vi "Backpressure Test.vi"() -> ()   [LabVIEW 2021]
uses:
  TypeDefs/Write Configuration.ctl
  TypeDefs/Read Configuration.ctl
  TypeDefs/Read Position.ctl
  TypeDefs/Data Element Details.ctl
  57e1f68e-aac2-4a5b-aa1d-bebc566d32eb.vi
  9744b0b2-8e27-4e4b-9bb7-f1c9ce8a1c96.vi
  07aec1d7-8ce0-4024-a95f-672f00c3de72.vi
  4385ff32-2761-4e03-bb1f-28e6c483433c.vi
  f7503771-80fd-45f4-b74f-3b2e92972461.vi
  c45c08b2-ea76-45d8-bd4a-0684d2e8d800.vi
  7eb9dc38-34d0-42a6-b102-5ea04e06049c.vi
  4e7c2fe8-0442-4db9-92fd-a364be716cb9.vi
  4ed2d6ae-5cba-444e-b9a2-7f82c0cf321a.vi
  ad8698de-81cd-4e11-8f1e-14e550fbdb4f.vi
  5ece5910-7f94-4528-9bc0-c785044b768d.vi
  f9d3fdbb-ee3c-4ad5-adeb-5751b16ba1b5.vi
  27686e40-44d3-4caa-b17a-767073325966.vi
  2cbba55c-0004-4c00-ad5c-760cc39579e2.vi
  0906a7d2-1e19-4f35-b09e-2fcf277513f2.vi
  7f108e34-9106-4d76-aec0-60a0699c295a.vi
  d49a2fac-eb09-4004-8c8e-5ff393d47214.vi
  3aa2fef3-6e97-4fad-b2b2-b9e5007bd319.vi
  66206acd-3047-480d-a13c-978b6dcd533f.vi
  a2f45c90-3ccc-4f15-aad7-08559cb123ac.vi
  32cec7b8-6370-43d4-931e-f60ddee9201a.vi
  63e088bb-fba7-44f9-b616-fb479035f017.vi
  b43ac5ef-eb88-421e-b33d-2ede57dd7442.vi
  e418e56f-4089-412c-bbf8-0d1a0f138b1a.vi
  e25f8ffa-7016-4157-92d2-29af65897e26.vi
  5e39a1b3-a940-464c-8f68-1595816f1c00.vi
  ac948e10-57ad-454e-bb7c-9577dd8c26ef.vi
  ffa58009-d41b-421a-8cf9-7a707b687784.vi
  8f16d32d-2386-471b-852e-c92f1fa65af2.vi
  57e1f68e-aac2-4a5b-aa1d-bebc566d32eb.vi/49b3dd2d-4579-4089-b72e-3f0875c862f2.vi
  SubVIs/Check Error.vi
  57e1f68e-aac2-4a5b-aa1d-bebc566d32eb.vi/1e2c93d0-55b0-4d6c-a9da-21395a664279.vi
  SubVIs/Get Backpressure Name.vi
  57e1f68e-aac2-4a5b-aa1d-bebc566d32eb.vi/7bb13226-97f3-4dcb-9346-06ec631a2876.vi
  SubVIs/Get dll Path.vi
  9744b0b2-8e27-4e4b-9bb7-f1c9ce8a1c96.vi/59915726-1e10-4578-8453-be1b9fd8d311.vi
  9744b0b2-8e27-4e4b-9bb7-f1c9ce8a1c96.vi/331f6ecb-7ec4-4931-b93d-4fbd8d66a851.vi
  07aec1d7-8ce0-4024-a95f-672f00c3de72.vi/3d5c1244-b460-4622-96d1-ee1e369932ac.vi
  Utilities/Get Size.vi
  07aec1d7-8ce0-4024-a95f-672f00c3de72.vi/b3361ac9-0b85-4d75-8feb-76d028d0c03f.vi
  SubVIs/Get Element Write Position.vi
  SubVIs/Notify Of New Write.vi
  f7503771-80fd-45f4-b74f-3b2e92972461.vi/49b3dd2d-4579-4089-b72e-3f0875c862f2.vi
  f7503771-80fd-45f4-b74f-3b2e92972461.vi/1e2c93d0-55b0-4d6c-a9da-21395a664279.vi
  f7503771-80fd-45f4-b74f-3b2e92972461.vi/7bb13226-97f3-4dcb-9346-06ec631a2876.vi
  c45c08b2-ea76-45d8-bd4a-0684d2e8d800.vi/59915726-1e10-4578-8453-be1b9fd8d311.vi
  c45c08b2-ea76-45d8-bd4a-0684d2e8d800.vi/331f6ecb-7ec4-4931-b93d-4fbd8d66a851.vi
  7eb9dc38-34d0-42a6-b102-5ea04e06049c.vi/3d5c1244-b460-4622-96d1-ee1e369932ac.vi
  7eb9dc38-34d0-42a6-b102-5ea04e06049c.vi/b3361ac9-0b85-4d75-8feb-76d028d0c03f.vi
  4ed2d6ae-5cba-444e-b9a2-7f82c0cf321a.vi/49b3dd2d-4579-4089-b72e-3f0875c862f2.vi
  4ed2d6ae-5cba-444e-b9a2-7f82c0cf321a.vi/1e2c93d0-55b0-4d6c-a9da-21395a664279.vi
  4ed2d6ae-5cba-444e-b9a2-7f82c0cf321a.vi/7bb13226-97f3-4dcb-9346-06ec631a2876.vi
  ad8698de-81cd-4e11-8f1e-14e550fbdb4f.vi/59915726-1e10-4578-8453-be1b9fd8d311.vi
  ad8698de-81cd-4e11-8f1e-14e550fbdb4f.vi/331f6ecb-7ec4-4931-b93d-4fbd8d66a851.vi
  5ece5910-7f94-4528-9bc0-c785044b768d.vi/3d5c1244-b460-4622-96d1-ee1e369932ac.vi
  5ece5910-7f94-4528-9bc0-c785044b768d.vi/b3361ac9-0b85-4d75-8feb-76d028d0c03f.vi
  27686e40-44d3-4caa-b17a-767073325966.vi/49b3dd2d-4579-4089-b72e-3f0875c862f2.vi
  27686e40-44d3-4caa-b17a-767073325966.vi/1e2c93d0-55b0-4d6c-a9da-21395a664279.vi
  27686e40-44d3-4caa-b17a-767073325966.vi/7bb13226-97f3-4dcb-9346-06ec631a2876.vi
  2cbba55c-0004-4c00-ad5c-760cc39579e2.vi/59915726-1e10-4578-8453-be1b9fd8d311.vi
  2cbba55c-0004-4c00-ad5c-760cc39579e2.vi/331f6ecb-7ec4-4931-b93d-4fbd8d66a851.vi
  0906a7d2-1e19-4f35-b09e-2fcf277513f2.vi/3d5c1244-b460-4622-96d1-ee1e369932ac.vi
  0906a7d2-1e19-4f35-b09e-2fcf277513f2.vi/b3361ac9-0b85-4d75-8feb-76d028d0c03f.vi
  d49a2fac-eb09-4004-8c8e-5ff393d47214.vi/49b3dd2d-4579-4089-b72e-3f0875c862f2.vi
  d49a2fac-eb09-4004-8c8e-5ff393d47214.vi/1e2c93d0-55b0-4d6c-a9da-21395a664279.vi
  d49a2fac-eb09-4004-8c8e-5ff393d47214.vi/7bb13226-97f3-4dcb-9346-06ec631a2876.vi
  3aa2fef3-6e97-4fad-b2b2-b9e5007bd319.vi/3d5c1244-b460-4622-96d1-ee1e369932ac.vi
  3aa2fef3-6e97-4fad-b2b2-b9e5007bd319.vi/b3361ac9-0b85-4d75-8feb-76d028d0c03f.vi
  a2f45c90-3ccc-4f15-aad7-08559cb123ac.vi/59915726-1e10-4578-8453-be1b9fd8d311.vi
  a2f45c90-3ccc-4f15-aad7-08559cb123ac.vi/331f6ecb-7ec4-4931-b93d-4fbd8d66a851.vi
  32cec7b8-6370-43d4-931e-f60ddee9201a.vi/bd07d5d9-1209-45ad-b636-9e9ab86132fb.vi
  32cec7b8-6370-43d4-931e-f60ddee9201a.vi/1e2c93d0-55b0-4d6c-a9da-21395a664279.vi
  32cec7b8-6370-43d4-931e-f60ddee9201a.vi/7bb13226-97f3-4dcb-9346-06ec631a2876.vi
  63e088bb-fba7-44f9-b616-fb479035f017.vi/331f6ecb-7ec4-4931-b93d-4fbd8d66a851.vi
  63e088bb-fba7-44f9-b616-fb479035f017.vi/5ce0d4cf-f921-42ba-b14c-c90f7f7611e4.vi
  b43ac5ef-eb88-421e-b33d-2ede57dd7442.vi/3d5c1244-b460-4622-96d1-ee1e369932ac.vi
  b43ac5ef-eb88-421e-b33d-2ede57dd7442.vi/b3361ac9-0b85-4d75-8feb-76d028d0c03f.vi
  e25f8ffa-7016-4157-92d2-29af65897e26.vi/bd07d5d9-1209-45ad-b636-9e9ab86132fb.vi
  e25f8ffa-7016-4157-92d2-29af65897e26.vi/1e2c93d0-55b0-4d6c-a9da-21395a664279.vi
  e25f8ffa-7016-4157-92d2-29af65897e26.vi/7bb13226-97f3-4dcb-9346-06ec631a2876.vi
  5e39a1b3-a940-464c-8f68-1595816f1c00.vi/331f6ecb-7ec4-4931-b93d-4fbd8d66a851.vi
  5e39a1b3-a940-464c-8f68-1595816f1c00.vi/5ce0d4cf-f921-42ba-b14c-c90f7f7611e4.vi
  ac948e10-57ad-454e-bb7c-9577dd8c26ef.vi/331f6ecb-7ec4-4931-b93d-4fbd8d66a851.vi
  ac948e10-57ad-454e-bb7c-9577dd8c26ef.vi/5ce0d4cf-f921-42ba-b14c-c90f7f7611e4.vi
  ffa58009-d41b-421a-8cf9-7a707b687784.vi/3d5c1244-b460-4622-96d1-ee1e369932ac.vi
  ffa58009-d41b-421a-8cf9-7a707b687784.vi/b3361ac9-0b85-4d75-8feb-76d028d0c03f.vi
  57e1f68e-aac2-4a5b-aa1d-bebc566d32eb.vi/1e2c93d0-55b0-4d6c-a9da-21395a664279.vi/49b3dd2d-4579-4089-b72e-3f0875c862f2.vi
  SubVIs/Wait For N Elements Available.vi
  SubVIs/Get Element Read Position.vi
  SubVIs/Set Element Read Position.vi
  f7503771-80fd-45f4-b74f-3b2e92972461.vi/1e2c93d0-55b0-4d6c-a9da-21395a664279.vi/49b3dd2d-4579-4089-b72e-3f0875c862f2.vi
  4ed2d6ae-5cba-444e-b9a2-7f82c0cf321a.vi/1e2c93d0-55b0-4d6c-a9da-21395a664279.vi/49b3dd2d-4579-4089-b72e-3f0875c862f2.vi
  27686e40-44d3-4caa-b17a-767073325966.vi/1e2c93d0-55b0-4d6c-a9da-21395a664279.vi/49b3dd2d-4579-4089-b72e-3f0875c862f2.vi
  d49a2fac-eb09-4004-8c8e-5ff393d47214.vi/1e2c93d0-55b0-4d6c-a9da-21395a664279.vi/49b3dd2d-4579-4089-b72e-3f0875c862f2.vi
  32cec7b8-6370-43d4-931e-f60ddee9201a.vi/1e2c93d0-55b0-4d6c-a9da-21395a664279.vi/49b3dd2d-4579-4089-b72e-3f0875c862f2.vi
  e25f8ffa-7016-4157-92d2-29af65897e26.vi/1e2c93d0-55b0-4d6c-a9da-21395a664279.vi/49b3dd2d-4579-4089-b72e-3f0875c862f2.vi
  <vilib>/Utility/error.llb/Trim Whitespace.vi
  <vilib>/string/Create NI GUID.vi
  SubVIs/Get Element Description Variant.vi
  <vilib>/Utility/error.llb/Error Cluster From Error Code.vi
  SubVIs/Get Element Info Variant.vi
  Core/Close.vi
  CIF_NI_CIPC.lvlib
panel:
  out "status":string
  out "pass":bool
  out "error out":errorcluster
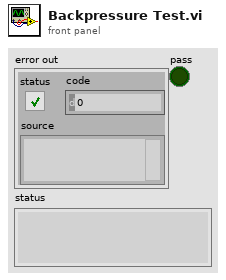
[diagram p1: front panel]
types:
  T1 = typedef "CIF_NI_CIPC.lvlib/Write Configuration.ctl" = cluster{"Prepend Array Size":bool, "Get Write Position":bool, "Notify Readers":bool}
  T2 = typedef "CIF_NI_CIPC.lvlib/Data Element Details.ctl" = cluster{"Bytes to Read":u32, "Element Offset":u32}
  T3 = typedef "CIF_NI_CIPC.lvlib/Read Configuration.ctl" = cluster{"Read Position":T4, "Element Offset":i32, "Prepend Array Size":bool, "Get Read Position":bool}
  T4 = typedef "CIF_NI_CIPC.lvlib/Read Position.ctl" = enum16{"Next", "Newest", "Oldest", "Next Available", "Absolute"}
  T5 = typedef "CIF_NI_CIPC.lvlib/Backpressure References.ctl" = cluster{"CIPC Reference":u64, "CIPC BP Reference":u64}
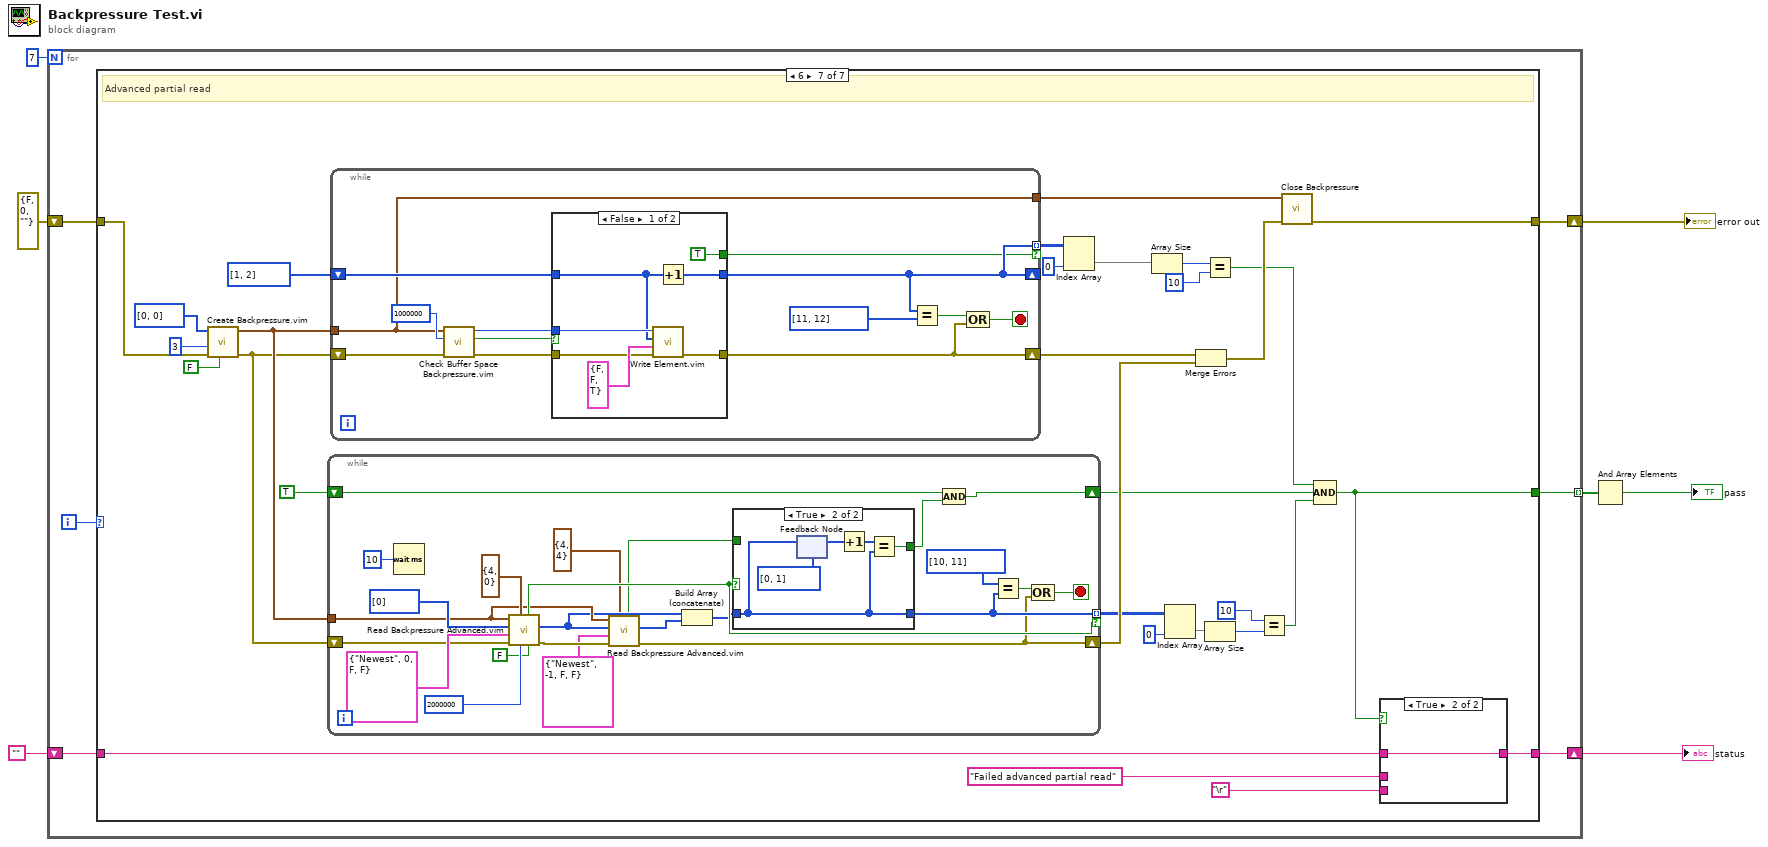
[diagram p0: block diagram]
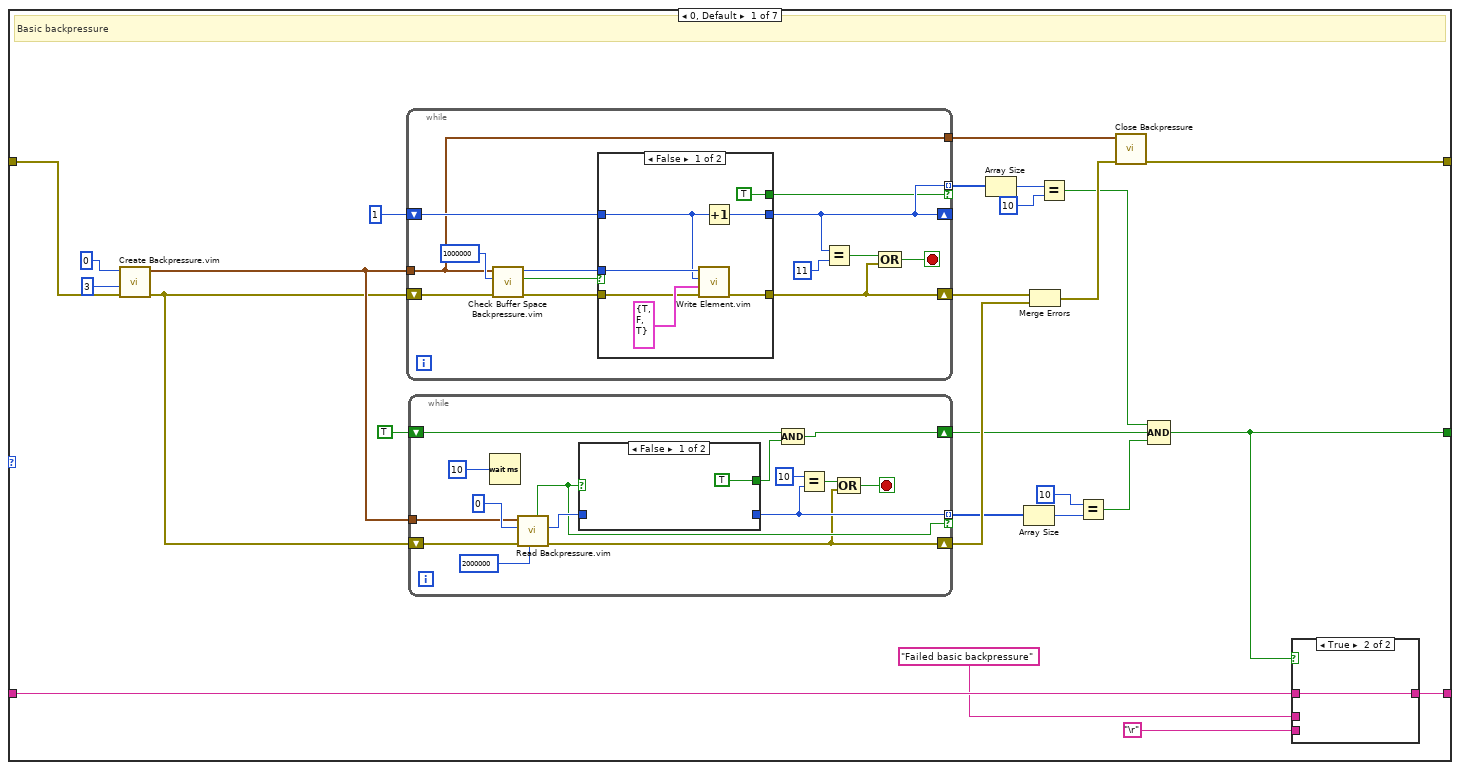
[diagram p2: hidden frame]
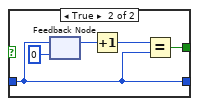
[diagram p3: hidden frame]
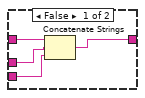
[diagram p5: hidden frame]
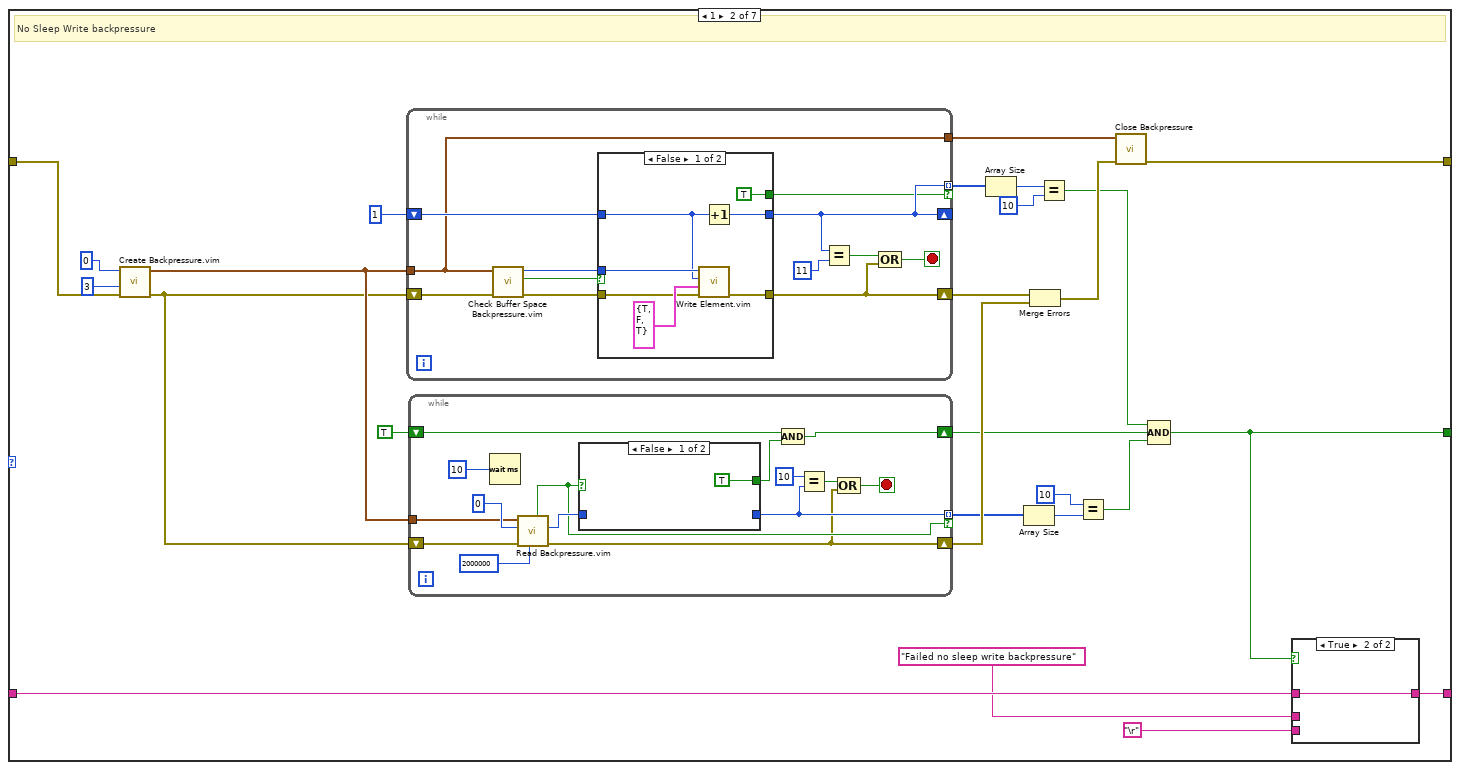
[diagram p6: hidden frame]
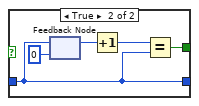
[diagram p7: hidden frame]
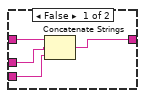
[diagram p9: hidden frame]
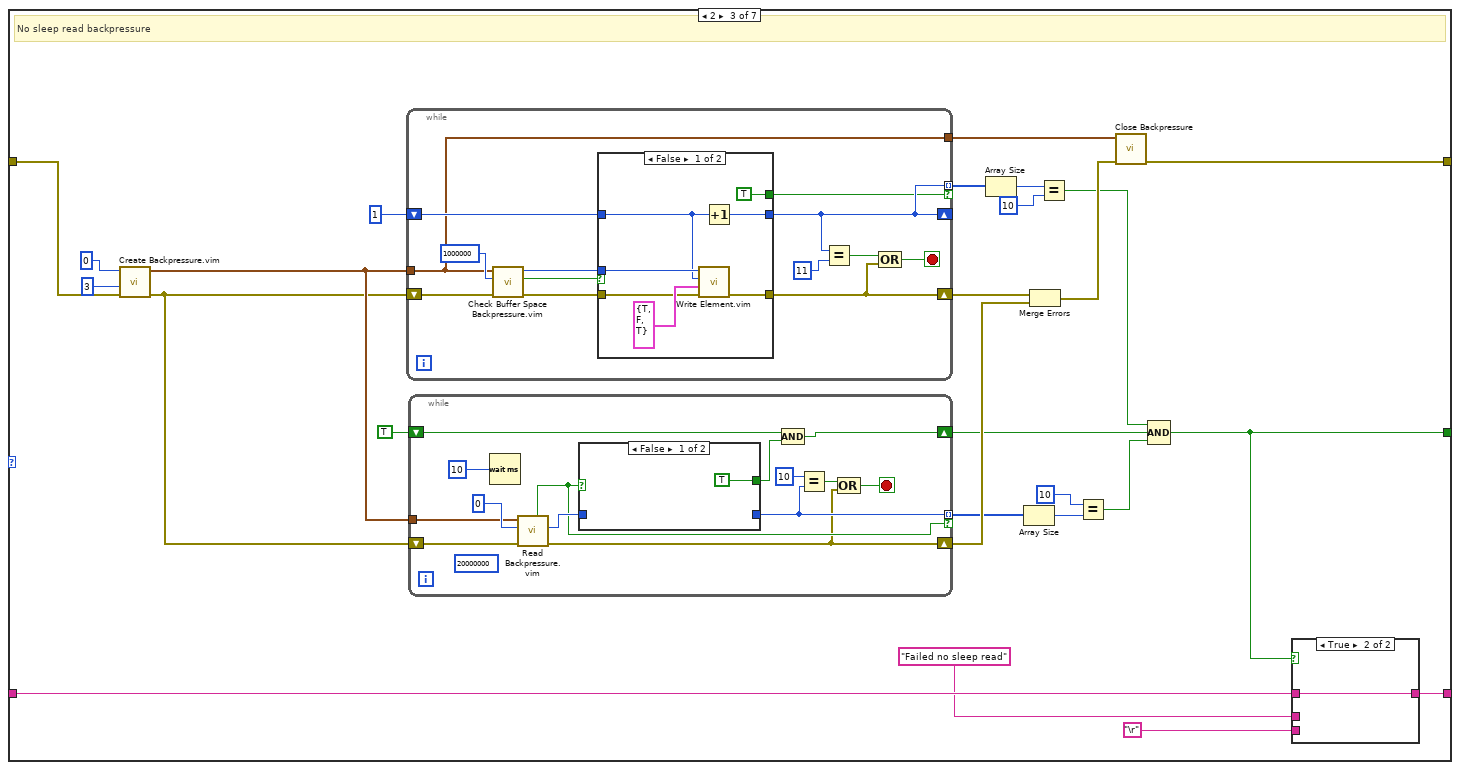
[diagram p10: hidden frame]
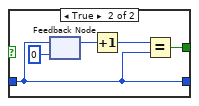
[diagram p11: hidden frame]
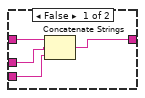
[diagram p13: hidden frame]
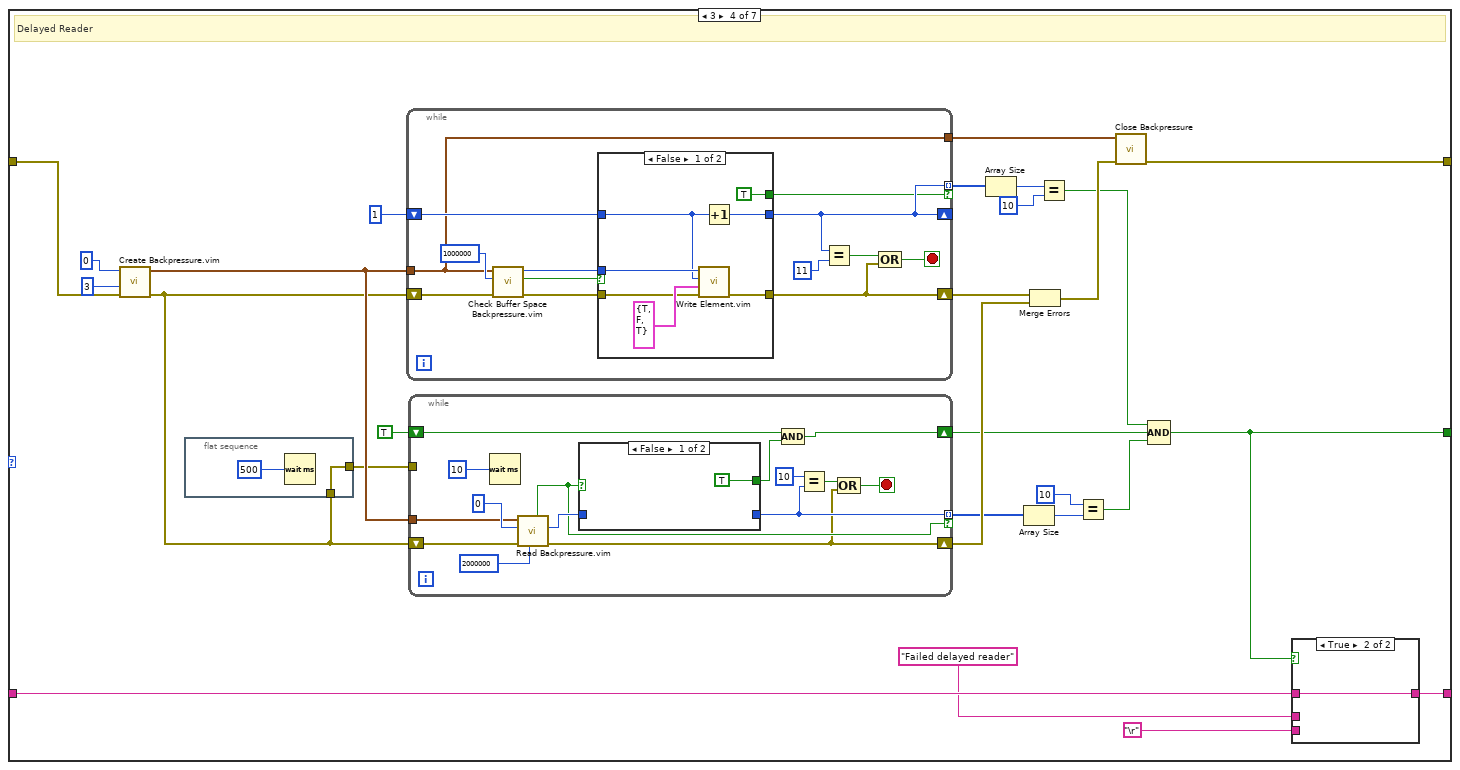
[diagram p14: hidden frame]
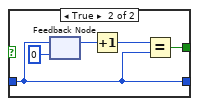
[diagram p15: hidden frame]
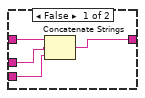
[diagram p17: hidden frame]
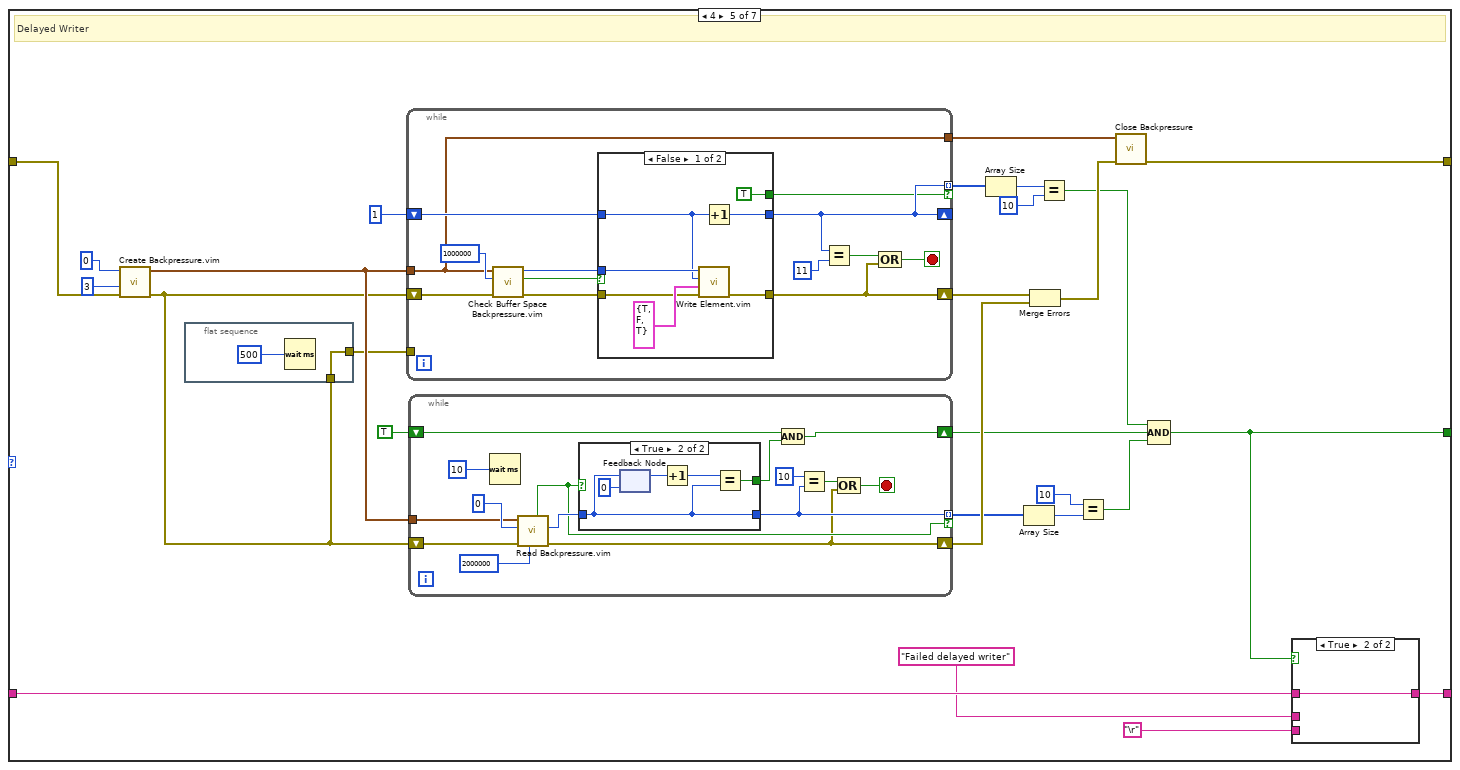
[diagram p18: hidden frame]
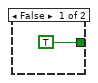
[diagram p19: hidden frame]
diagram:
  n1 = for {
    N: 7 -> [_]
    tunnel: [w13] -> w7 mode=indexing
    shift-right: [w10] -> w1
    shift-left: "" -> [w11]
    shift-right: [w9] -> w2
    shift-left: errorcluster {"status"=FALSE, "code"=0, "source"=""} ("error out") -> [w8]
    i -> [w12]
    n2 = case shown="6" w12 {
      tunnel: [w18 w92 w165 w240 w317 w400 w481] -> w13
      tunnel: w11 -> [w39 w113 w186 w260 w337 w418 w499]
      tunnel: [w38 w112 w185 w259 w336 w417 w498] -> w10
      tunnel: [w28 w102 w175 w249 w326 w408 w489] -> w9
      tunnel: w8 -> [w29 w103 w176 w250 w327 w409 w490]
      frame 0, Default {
        # "Basic backpressure"
        n3 = call "Create Backpressure.vim"("error in (no error)"=w29, "Buffer Size N (2^N)"=u8 3, "Data Type"=0) -> ("error out"=w24:errorcluster, "CIPC BP References"=w25:T5)  [unwired: 5 in, 2 out]
        n4 = while {
          tunnel: w25 -> [w61]
          shift-right: [w66] -> w33
          shift-left: w24 -> [w73]
          shift-right: [w63] -> _
          shift-left: 1 ("Data out") -> [w64]
          tunnel: [w63] -> w17 mode=indexing if=w62
          tunnel: [w61] -> w26
          stop <- w65 stop-if-true
          n5 = call "Check Buffer Space Backpressure.vim"("error in (no error)"=w73, "Timeout (ns)"=i64 1000000, "CIPC BP References in"=w61) -> ("error out"=w72:errorcluster, "Timeout"=w70:bool, "CIPC Reference out"=w71:u64)  [unwired: 6 in]
          n6 = case shown="False" w70 {
            tunnel: w71 -> [w79 _]
            tunnel: w72 -> [w78 w82]
            tunnel: [w77 w82] -> w66
            tunnel: w64 -> [w76 w81]
            tunnel: [w75 w81] -> w63
            tunnel: [TRUE _] -> w62
            frame False {
              n7 = call "Write Element.vim"("error in (no error)"=w78, "Write Configuration"=T1 {"Prepend Array Size"=TRUE, "Get Write Position"=FALSE, "Notify Readers"=TRUE}, "Data in"=w76, "CIPC Reference in"=w79) -> ("error out"=w77:errorcluster)  [unwired: 4 in, 3 out]
              n8 = Increment(x=w76) -> (x+1=w75:i32)
            }
            frame True {
              # "Timeout"
            }
          }
          n9 = Equal?(x=w63, y=11) -> (x = y?=w67:bool)
          n10 = Compound Arithmetic op=OR(w67, w66) -> (w65:bool)
        }
        n11 = while {
          shift-right: [w49] -> w20
          shift-left: TRUE -> [w53]
          shift-right: [w44] -> w34
          shift-left: w24 -> [w51]
          tunnel: [w47] -> w23 mode=indexing if=w48
          tunnel: w25 -> [w40]
          stop <- w43 stop-if-true
          n12 = Wait (ms)(milliseconds to wait=u32 10) -> ()  [unwired: 1 out]
          n13 = call "Read Backpressure.vim"("Timeout (ns)"=2000000, "error in (no error)"=w51, "Data in"=0, "CIPC BP References in"=w40) -> ("error out"=w44:errorcluster, "Data out"=w50:i32, "Success"=w48:bool)  [unwired: 3 in, 2 out]
          n14 = case shown="False" w48 {
            tunnel: w50 -> [_ w56]
            tunnel: [TRUE w57] -> w52
            tunnel: [_ w56] -> w47
            frame False {
            }
            frame True {
              n15 = feedback #1(0 ("Data out")) -> (w59:i32)
              n16 = feedback-in #1(w56) -> ()
              n17 = Increment(x=w59) -> (x+1=w58:i32)
              n18 = Equal?(x=w58, y=w56) -> (x = y?=w57:bool)
            }
          }
          n19 = Compound Arithmetic op=AND(w53, w52) -> (w49:bool)
          n20 = Equal?(x=10, y=w47) -> (x = y?=w45:bool)
          n21 = Compound Arithmetic op=OR(w45, w44) -> (w43:bool)
        }
        n22 = Array Size(array=w17) -> (size(s)=w16:i32)
        n23 = Array Size(array=w23) -> (size(s)=w22:i32)
        n24 = Merge Errors(w33, w34) -> (w35:errorcluster)
        n25 = Equal?(x=w16, y=10 ("x")) -> (x = y?=w14:bool)
        n26 = Equal?(x=10, y=w22) -> (x = y?=w19:bool)
        n27 = call "Close Backpressure.vi"("error in (no error)"=w35, "CIPC BP References in"=w26) -> ("error out"=w28:errorcluster)  [unwired: 9 in]
        n28 = Compound Arithmetic op=AND(w14, w20, w19) -> (w18:bool)
        n29 = case shown="True" w18 {
          tunnel: w39 -> [w86 w87]
          tunnel: [w83 w87] -> w38
          tunnel: "Failed basic backpressure" -> [w85 _]
          tunnel: "\r" -> [w84 _]
          frame False {
            n30 = Concatenate Strings(w86, w85, w84) -> (w83:string)
          }
          frame True {
          }
        }
      }
      frame 1 {
        # "No Sleep Write backpressure"
        n31 = call "Create Backpressure.vim"("error in (no error)"=w103, "Buffer Size N (2^N)"=u8 3, "Data Type"=0) -> ("error out"=w98:errorcluster, "CIPC BP References"=w99:T5)  [unwired: 5 in, 2 out]
        n32 = while {
          tunnel: w99 -> [w135]
          shift-right: [w140] -> w107
          shift-left: w98 -> [w146]
          shift-right: [w137] -> _
          shift-left: 1 ("Data out") -> [w138]
          tunnel: [w137] -> w91 mode=indexing if=w136
          tunnel: [w135] -> w100
          stop <- w139 stop-if-true
          n33 = call "Check Buffer Space Backpressure.vim"("error in (no error)"=w146, "CIPC BP References in"=w135) -> ("error out"=w145:errorcluster, "Timeout"=w143:bool, "CIPC Reference out"=w144:u64)  [unwired: 7 in]
          n34 = case shown="False" w143 {
            tunnel: w144 -> [w152 _]
            tunnel: w145 -> [w151 w155]
            tunnel: [w150 w155] -> w140
            tunnel: w138 -> [w149 w154]
            tunnel: [w148 w154] -> w137
            tunnel: [TRUE _] -> w136
            frame False {
              n35 = call "Write Element.vim"("error in (no error)"=w151, "Write Configuration"=T1 {"Prepend Array Size"=TRUE, "Get Write Position"=FALSE, "Notify Readers"=TRUE}, "Data in"=w149, "CIPC Reference in"=w152) -> ("error out"=w150:errorcluster)  [unwired: 4 in, 3 out]
              n36 = Increment(x=w149) -> (x+1=w148:i32)
            }
            frame True {
              # "Timeout"
            }
          }
          n37 = Equal?(x=w137, y=11) -> (x = y?=w141:bool)
          n38 = Compound Arithmetic op=OR(w141, w140) -> (w139:bool)
        }
        n39 = while {
          shift-right: [w123] -> w94
          shift-left: TRUE -> [w127]
          shift-right: [w118] -> w108
          shift-left: w98 -> [w125]
          tunnel: [w121] -> w97 mode=indexing if=w122
          tunnel: w99 -> [w114]
          stop <- w117 stop-if-true
          n40 = Wait (ms)(milliseconds to wait=u32 10) -> ()  [unwired: 1 out]
          n41 = call "Read Backpressure.vim"("Timeout (ns)"=2000000, "error in (no error)"=w125, "Data in"=0, "CIPC BP References in"=w114) -> ("error out"=w118:errorcluster, "Data out"=w124:i32, "Success"=w122:bool)  [unwired: 3 in, 2 out]
          n42 = case shown="False" w122 {
            tunnel: w124 -> [_ w130]
            tunnel: [TRUE w131] -> w126
            tunnel: [_ w130] -> w121
            frame False {
            }
            frame True {
              n43 = feedback #2(0 ("Data out")) -> (w133:i32)
              n44 = feedback-in #2(w130) -> ()
              n45 = Increment(x=w133) -> (x+1=w132:i32)
              n46 = Equal?(x=w132, y=w130) -> (x = y?=w131:bool)
            }
          }
          n47 = Compound Arithmetic op=AND(w127, w126) -> (w123:bool)
          n48 = Equal?(x=10, y=w121) -> (x = y?=w119:bool)
          n49 = Compound Arithmetic op=OR(w119, w118) -> (w117:bool)
        }
        n50 = Array Size(array=w91) -> (size(s)=w90:i32)
        n51 = Array Size(array=w97) -> (size(s)=w96:i32)
        n52 = Merge Errors(w107, w108) -> (w109:errorcluster)
        n53 = Equal?(x=w90, y=10 ("x")) -> (x = y?=w88:bool)
        n54 = Equal?(x=10, y=w96) -> (x = y?=w93:bool)
        n55 = call "Close Backpressure.vi"("error in (no error)"=w109, "CIPC BP References in"=w100) -> ("error out"=w102:errorcluster)  [unwired: 9 in]
        n56 = Compound Arithmetic op=AND(w88, w94, w93) -> (w92:bool)
        n57 = case shown="True" w92 {
          tunnel: w113 -> [w159 w160]
          tunnel: [w156 w160] -> w112
          tunnel: "Failed no sleep write backpressure" -> [w158 _]
          tunnel: "\r" -> [w157 _]
          frame False {
            n58 = Concatenate Strings(w159, w158, w157) -> (w156:string)
          }
          frame True {
          }
        }
      }
      frame 2 {
        # "No sleep read backpressure"
        n59 = call "Create Backpressure.vim"("error in (no error)"=w176, "Buffer Size N (2^N)"=u8 3, "Data Type"=0) -> ("error out"=w171:errorcluster, "CIPC BP References"=w172:T5)  [unwired: 5 in, 2 out]
        n60 = while {
          tunnel: w172 -> [w207]
          shift-right: [w212] -> w180
          shift-left: w171 -> [w219]
          shift-right: [w209] -> _
          shift-left: 1 ("Data out") -> [w210]
          tunnel: [w209] -> w164 mode=indexing if=w208
          tunnel: [w207] -> w173
          stop <- w211 stop-if-true
          n61 = call "Check Buffer Space Backpressure.vim"("error in (no error)"=w219, "Timeout (ns)"=i64 1000000, "CIPC BP References in"=w207) -> ("error out"=w218:errorcluster, "Timeout"=w216:bool, "CIPC Reference out"=w217:u64)  [unwired: 6 in]
          n62 = case shown="False" w216 {
            tunnel: w217 -> [w225 _]
            tunnel: w218 -> [w224 w228]
            tunnel: [w223 w228] -> w212
            tunnel: w210 -> [w222 w227]
            tunnel: [w221 w227] -> w209
            tunnel: [TRUE _] -> w208
            frame False {
              n63 = call "Write Element.vim"("error in (no error)"=w224, "Write Configuration"=T1 {"Prepend Array Size"=TRUE, "Get Write Position"=FALSE, "Notify Readers"=TRUE}, "Data in"=w222, "CIPC Reference in"=w225) -> ("error out"=w223:errorcluster)  [unwired: 4 in, 3 out]
              n64 = Increment(x=w222) -> (x+1=w221:i32)
            }
            frame True {
              # "Timeout"
            }
          }
          n65 = Equal?(x=w209, y=11) -> (x = y?=w213:bool)
          n66 = Compound Arithmetic op=OR(w213, w212) -> (w211:bool)
        }
        n67 = while {
          shift-right: [w195] -> w167
          shift-left: TRUE -> [w199]
          shift-right: [w190] -> w181
          shift-left: w171 -> [w197]
          tunnel: [w193] -> w170 mode=indexing if=w194
          tunnel: w172 -> [w187]
          stop <- w189 stop-if-true
          (unwired) 20000000
          n68 = Wait (ms)(milliseconds to wait=u32 10) -> ()  [unwired: 1 out]
          n69 = call "Read Backpressure.vim"("error in (no error)"=w197, "Data in"=0, "CIPC BP References in"=w187) -> ("error out"=w190:errorcluster, "Data out"=w196:i32, "Success"=w194:bool)  [unwired: 4 in, 2 out]
          n70 = case shown="False" w194 {
            tunnel: w196 -> [_ w202]
            tunnel: [TRUE w203] -> w198
            tunnel: [_ w202] -> w193
            frame False {
            }
            frame True {
              n71 = feedback #3(0 ("Data out")) -> (w205:i32)
              n72 = feedback-in #3(w202) -> ()
              n73 = Increment(x=w205) -> (x+1=w204:i32)
              n74 = Equal?(x=w204, y=w202) -> (x = y?=w203:bool)
            }
          }
          n75 = Compound Arithmetic op=AND(w199, w198) -> (w195:bool)
          n76 = Equal?(x=10, y=w193) -> (x = y?=w191:bool)
          n77 = Compound Arithmetic op=OR(w191, w190) -> (w189:bool)
        }
        n78 = Array Size(array=w164) -> (size(s)=w163:i32)
        n79 = Array Size(array=w170) -> (size(s)=w169:i32)
        n80 = Merge Errors(w180, w181) -> (w182:errorcluster)
        n81 = Equal?(x=w163, y=10 ("x")) -> (x = y?=w161:bool)
        n82 = Equal?(x=10, y=w169) -> (x = y?=w166:bool)
        n83 = call "Close Backpressure.vi"("error in (no error)"=w182, "CIPC BP References in"=w173) -> ("error out"=w175:errorcluster)  [unwired: 9 in]
        n84 = Compound Arithmetic op=AND(w161, w167, w166) -> (w165:bool)
        n85 = case shown="True" w165 {
          tunnel: w186 -> [w232 w233]
          tunnel: [w229 w233] -> w185
          tunnel: "Failed no sleep read" -> [w231 _]
          tunnel: "\r" -> [w230 _]
          frame False {
            n86 = Concatenate Strings(w232, w231, w230) -> (w229:string)
          }
          frame True {
          }
        }
      }
      frame 3 {
        # "Delayed Reader"
        n87 = call "Create Backpressure.vim"("error in (no error)"=w250, "Buffer Size N (2^N)"=u8 3, "Data Type"=0) -> ("error out"=w235:errorcluster, "CIPC BP References"=w246:T5)  [unwired: 5 in, 2 out]
        n88 = flat-sequence {
          tunnel: w235 -> [w261]
          tunnel: [w261] -> w234
          frame #0 {
            n89 = Wait (ms)(milliseconds to wait=u32 500) -> ()  [unwired: 1 out]
          }
        }
        n90 = while {
          tunnel: w246 -> [w284]
          shift-right: [w289] -> w254
          shift-left: w235 -> [w296]
          shift-right: [w286] -> _
          shift-left: 1 ("Data out") -> [w287]
          tunnel: [w286] -> w239 mode=indexing if=w285
          tunnel: [w284] -> w247
          stop <- w288 stop-if-true
          n91 = call "Check Buffer Space Backpressure.vim"("error in (no error)"=w296, "Timeout (ns)"=i64 1000000, "CIPC BP References in"=w284) -> ("error out"=w295:errorcluster, "Timeout"=w293:bool, "CIPC Reference out"=w294:u64)  [unwired: 6 in]
          n92 = case shown="False" w293 {
            tunnel: w294 -> [w302 _]
            tunnel: w295 -> [w301 w305]
            tunnel: [w300 w305] -> w289
            tunnel: w287 -> [w299 w304]
            tunnel: [w298 w304] -> w286
            tunnel: [TRUE _] -> w285
            frame False {
              n93 = call "Write Element.vim"("error in (no error)"=w301, "Write Configuration"=T1 {"Prepend Array Size"=TRUE, "Get Write Position"=FALSE, "Notify Readers"=TRUE}, "Data in"=w299, "CIPC Reference in"=w302) -> ("error out"=w300:errorcluster)  [unwired: 4 in, 3 out]
              n94 = Increment(x=w299) -> (x+1=w298:i32)
            }
            frame True {
              # "Timeout"
            }
          }
          n95 = Equal?(x=w286, y=11) -> (x = y?=w290:bool)
          n96 = Compound Arithmetic op=OR(w290, w289) -> (w288:bool)
        }
        n97 = while {
          shift-right: [w272] -> w242
          shift-left: TRUE -> [w276]
          shift-right: [w267] -> w255
          shift-left: w235 -> [w274]
          tunnel: [w270] -> w245 mode=indexing if=w271
          tunnel: w246 -> [w263]
          tunnel: w234 -> [_]
          stop <- w266 stop-if-true
          n98 = Wait (ms)(milliseconds to wait=u32 10) -> ()  [unwired: 1 out]
          n99 = call "Read Backpressure.vim"("Timeout (ns)"=2000000, "error in (no error)"=w274, "Data in"=0, "CIPC BP References in"=w263) -> ("error out"=w267:errorcluster, "Data out"=w273:i32, "Success"=w271:bool)  [unwired: 3 in, 2 out]
          n100 = case shown="False" w271 {
            tunnel: w273 -> [_ w279]
            tunnel: [TRUE w280] -> w275
            tunnel: [_ w279] -> w270
            frame False {
            }
            frame True {
              n101 = feedback #4(0 ("Data out")) -> (w282:i32)
              n102 = feedback-in #4(w279) -> ()
              n103 = Increment(x=w282) -> (x+1=w281:i32)
              n104 = Equal?(x=w281, y=w279) -> (x = y?=w280:bool)
            }
          }
          n105 = Compound Arithmetic op=AND(w276, w275) -> (w272:bool)
          n106 = Equal?(x=10, y=w270) -> (x = y?=w268:bool)
          n107 = Compound Arithmetic op=OR(w268, w267) -> (w266:bool)
        }
        n108 = Array Size(array=w239) -> (size(s)=w238:i32)
        n109 = Array Size(array=w245) -> (size(s)=w244:i32)
        n110 = Merge Errors(w254, w255) -> (w256:errorcluster)
        n111 = Equal?(x=w238, y=10 ("x")) -> (x = y?=w236:bool)
        n112 = Equal?(x=10, y=w244) -> (x = y?=w241:bool)
        n113 = call "Close Backpressure.vi"("error in (no error)"=w256, "CIPC BP References in"=w247) -> ("error out"=w249:errorcluster)  [unwired: 9 in]
        n114 = Compound Arithmetic op=AND(w236, w242, w241) -> (w240:bool)
        n115 = case shown="True" w240 {
          tunnel: w260 -> [w309 w310]
          tunnel: [w306 w310] -> w259
          tunnel: "Failed delayed reader" -> [w308 _]
          tunnel: "\r" -> [w307 _]
          frame False {
            n116 = Concatenate Strings(w309, w308, w307) -> (w306:string)
          }
          frame True {
          }
        }
      }
      frame 4 {
        # "Delayed Writer"
        n117 = call "Create Backpressure.vim"("error in (no error)"=w327, "Buffer Size N (2^N)"=u8 3, "Data Type"=0) -> ("error out"=w312:errorcluster, "CIPC BP References"=w323:T5)  [unwired: 5 in, 2 out]
        n118 = flat-sequence {
          tunnel: w312 -> [w338]
          tunnel: [w338] -> w311
          frame #0 {
            n119 = Wait (ms)(milliseconds to wait=u32 500) -> ()  [unwired: 1 out]
          }
        }
        n120 = while {
          tunnel: w323 -> [w361]
          shift-right: [w366] -> w331
          shift-left: w312 -> [w373]
          shift-right: [w363] -> _
          shift-left: 1 ("Data out") -> [w364]
          tunnel: [w363] -> w316 mode=indexing if=w362
          tunnel: [w361] -> w324
          tunnel: w311 -> [_]
          stop <- w365 stop-if-true
          n121 = call "Check Buffer Space Backpressure.vim"("error in (no error)"=w373, "Timeout (ns)"=i64 1000000, "CIPC BP References in"=w361) -> ("error out"=w372:errorcluster, "Timeout"=w370:bool, "CIPC Reference out"=w371:u64)  [unwired: 6 in]
          n122 = case shown="False" w370 {
            tunnel: w371 -> [w379 _]
            tunnel: w372 -> [w378 w382]
            tunnel: [w377 w382] -> w366
            tunnel: w364 -> [w376 w381]
            tunnel: [w375 w381] -> w363
            tunnel: [TRUE _] -> w362
            frame False {
              n123 = call "Write Element.vim"("error in (no error)"=w378, "Write Configuration"=T1 {"Prepend Array Size"=TRUE, "Get Write Position"=FALSE, "Notify Readers"=TRUE}, "Data in"=w376, "CIPC Reference in"=w379) -> ("error out"=w377:errorcluster)  [unwired: 4 in, 3 out]
              n124 = Increment(x=w376) -> (x+1=w375:i32)
            }
            frame True {
              # "Timeout"
            }
          }
          n125 = Equal?(x=w363, y=11) -> (x = y?=w367:bool)
          n126 = Compound Arithmetic op=OR(w367, w366) -> (w365:bool)
        }
        n127 = while {
          shift-right: [w349] -> w319
          shift-left: TRUE -> [w353]
          shift-right: [w344] -> w332
          shift-left: w312 -> [w351]
          tunnel: [w347] -> w322 mode=indexing if=w348
          tunnel: w323 -> [w340]
          stop <- w343 stop-if-true
          n128 = Wait (ms)(milliseconds to wait=u32 10) -> ()  [unwired: 1 out]
          n129 = call "Read Backpressure.vim"("Timeout (ns)"=2000000, "error in (no error)"=w351, "Data in"=0, "CIPC BP References in"=w340) -> ("error out"=w344:errorcluster, "Data out"=w350:i32, "Success"=w348:bool)  [unwired: 3 in, 2 out]
          n130 = case shown="True" w348 {
            tunnel: w350 -> [_ w356]
            tunnel: [TRUE w357] -> w352
            tunnel: [_ w356] -> w347
            frame False {
            }
            frame True {
              n131 = feedback #5(0 ("Data out")) -> (w359:i32)
              n132 = feedback-in #5(w356) -> ()
              n133 = Increment(x=w359) -> (x+1=w358:i32)
              n134 = Equal?(x=w358, y=w356) -> (x = y?=w357:bool)
            }
          }
          n135 = Compound Arithmetic op=AND(w353, w352) -> (w349:bool)
          n136 = Equal?(x=10, y=w347) -> (x = y?=w345:bool)
          n137 = Compound Arithmetic op=OR(w345, w344) -> (w343:bool)
        }
        n138 = Array Size(array=w316) -> (size(s)=w315:i32)
        n139 = Array Size(array=w322) -> (size(s)=w321:i32)
        n140 = Merge Errors(w331, w332) -> (w333:errorcluster)
        n141 = Equal?(x=w315, y=10 ("x")) -> (x = y?=w313:bool)
        n142 = Equal?(x=10, y=w321) -> (x = y?=w318:bool)
        n143 = call "Close Backpressure.vi"("error in (no error)"=w333, "CIPC BP References in"=w324) -> ("error out"=w326:errorcluster)  [unwired: 9 in]
        n144 = Compound Arithmetic op=AND(w313, w319, w318) -> (w317:bool)
        n145 = case shown="True" w317 {
          tunnel: w337 -> [w386 w387]
          tunnel: [w383 w387] -> w336
          tunnel: "Failed delayed writer" -> [w385 _]
          tunnel: "\r" -> [w384 _]
          frame False {
            n146 = Concatenate Strings(w386, w385, w384) -> (w383:string)
          }
          frame True {
          }
        }
      }
      frame 5 {
        # "Advanced full read"
        n147 = call "Create Backpressure.vim"("Prepend Array Size"=FALSE, "error in (no error)"=w409, "Buffer Size N (2^N)"=u8 3, "Data Type"=i32[] [0, 0]) -> ("error out"=w405:errorcluster, "CIPC BP References"=w406:T5)  [unwired: 4 in, 2 out]
        n148 = while {
          shift-right: [w432] -> w402
          shift-left: TRUE -> [w434]
          shift-right: [w423] -> w413
          shift-left: w405 -> [w425]
          tunnel: [w431] -> w392 mode=indexing if=w420
          tunnel: w406 -> [w427]
          stop <- w429 stop-if-true
          n149 = Wait (ms)(milliseconds to wait=u32 10) -> ()  [unwired: 1 out]
          n150 = call "Read Backpressure Advanced.vim"("Timeout (ns)"=2000000, "Data Element"=T2 {"Bytes to Read"=8, "Element Offset"=0}, "error in (no error)"=w425, "Read Configuration"=T3 {"Read Position"=enum."Newest", "Element Offset"=0, "Prepend Array Size"=FALSE, "Get Read Position"=FALSE}, "Data in"=i32[] [0, 0], "CIPC BP References in"=w427) -> ("error out"=w423:errorcluster, "Data out"=w422:i32[], "Success"=w420:bool)  [unwired: 1 in, 2 out]
          n151 = case shown="True" w420 {
            tunnel: w422 -> [_ w438]
            tunnel: [TRUE w439] -> w433
            tunnel: [_ w438] -> w431
            frame False {
            }
            frame True {
              n152 = feedback #6(i32[] [0, 0]) -> (w441:i32[])
              n153 = feedback-in #6(w438) -> ()
              n154 = Increment(x=w441) -> (x+1=w440:i32[])
              n155 = Equal?(x=w440, y=w438) -> (x = y?=w439:bool)
            }
          }
          n156 = Compound Arithmetic op=AND(w434, w433) -> (w432:bool)
          n157 = Equal?(x=i32[] [10, 10], y=w431) -> (x = y?=w430:bool)
          n158 = Compound Arithmetic op=OR(w430, w423) -> (w429:bool)
        }
        n159 = while {
          tunnel: w406 -> [w443]
          shift-right: [w448] -> w412
          shift-left: w405 -> [w454]
          shift-right: [w445] -> _
          shift-left: i32[] [1, 1] -> [w446]
          tunnel: [w445] -> w394 mode=indexing if=w444
          tunnel: [w443] -> w407
          stop <- w447 stop-if-true
          n160 = call "Check Buffer Space Backpressure.vim"("error in (no error)"=w454, "Timeout (ns)"=i64 1000000, "CIPC BP References in"=w443) -> ("error out"=w453:errorcluster, "Timeout"=w451:bool, "CIPC Reference out"=w452:u64)  [unwired: 6 in]
          n161 = case shown="False" w451 {
            tunnel: w452 -> [w460 _]
            tunnel: w453 -> [w459 w463]
            tunnel: [w458 w463] -> w448
            tunnel: w446 -> [w457 w462]
            tunnel: [w456 w462] -> w445
            tunnel: [TRUE _] -> w444
            frame False {
              n162 = call "Write Element.vim"("error in (no error)"=w459, "Write Configuration"=T1 {"Prepend Array Size"=FALSE, "Get Write Position"=FALSE, "Notify Readers"=TRUE}, "Data in"=w457, "CIPC Reference in"=w460) -> ("error out"=w458:errorcluster)  [unwired: 4 in, 3 out]
              n163 = Increment(x=w457) -> (x+1=w456:i32[])
            }
            frame True {
              # "Timeout"
            }
          }
          n164 = Equal?(x=w445, y=i32[] [11, 11]) -> (x = y?=w449:bool)
          n165 = Compound Arithmetic op=OR(w449, w448) -> (w447:bool)
        }
        n166 = Index Array(array=w394, index (col)=0 ("disabled index (col)")) -> (element=w393:i32[])  [unwired: 1 in]
        n167 = Array Size(array=w393) -> (size(s)=w399:i32)
        n168 = Index Array(array=w392, index (col)=0 ("disabled index (col)")) -> (element=w391:i32[])  [unwired: 1 in]
        n169 = Merge Errors(w412, w413) -> (w414:errorcluster)
        n170 = Equal?(x=w399, y=10 ("x")) -> (x = y?=w397:bool)
        n171 = Array Size(array=w391) -> (size(s)=w404:i32)
        n172 = Equal?(x=10, y=w404) -> (x = y?=w401:bool)
        n173 = call "Close Backpressure.vi"("error in (no error)"=w414, "CIPC BP References in"=w407) -> ("error out"=w408:errorcluster)  [unwired: 9 in]
        n174 = Compound Arithmetic op=AND(w397, w402, w401) -> (w400:bool)
        n175 = case shown="True" w400 {
          tunnel: w418 -> [w467 w468]
          tunnel: [w464 w468] -> w417
          tunnel: "Failed advanced full read" -> [w466 _]
          tunnel: "\r" -> [w465 _]
          frame False {
            n176 = Concatenate Strings(w467, w466, w465) -> (w464:string)
          }
          frame True {
          }
        }
      }
      frame 6 {
        # "Advanced partial read"
        n177 = call "Create Backpressure.vim"("Prepend Array Size"=FALSE, "error in (no error)"=w490, "Buffer Size N (2^N)"=u8 3, "Data Type"=i32[] [0, 0]) -> ("error out"=w486:errorcluster, "CIPC BP References"=w487:T5)  [unwired: 4 in, 2 out]
        n178 = while {
          shift-right: [w520] -> w483
          shift-left: TRUE -> [w522]
          shift-right: [w505] -> w494
          shift-left: w486 -> [w514]
          tunnel: [w519] -> w473 mode=indexing if=w511
          tunnel: w487 -> [w509]
          stop <- w517 stop-if-true
          n179 = Wait (ms)(milliseconds to wait=u32 10) -> ()  [unwired: 1 out]
          n180 = call "Read Backpressure Advanced.vim"("Last Read"=FALSE, "Timeout (ns)"=2000000, "Data Element"=T2 {"Bytes to Read"=4, "Element Offset"=0}, "error in (no error)"=w514, "Read Configuration"=T3 {"Read Position"=enum."Newest", "Element Offset"=0, "Prepend Array Size"=FALSE, "Get Read Position"=FALSE}, "Data in"=i32[] [0], "CIPC BP References in"=w509) -> ("error out"=w508:errorcluster, "Data out"=w506:i32[], "Success"=w511:bool)  [unwired: 2 out]
          n181 = call "Read Backpressure Advanced.vim"("Data Element"=T2 {"Bytes to Read"=4, "Element Offset"=4}, "error in (no error)"=w508, "Read Configuration"=T3 {"Read Position"=enum."Newest", "Element Offset"=-1, "Prepend Array Size"=FALSE, "Get Read Position"=FALSE}, "Data in"=w506, "CIPC BP References in"=w509) -> ("error out"=w505:errorcluster, "Data out"=w507:i32[], "Success"=w500:bool)  [unwired: 2 in, 2 out]
          n182 = Build Array (concatenate)(w506, w507) -> (w504:i32[])
          n183 = case shown="True" w511 {
            tunnel: w504 -> [_ w526]
            tunnel: [TRUE w527] -> w521
            tunnel: [_ w526] -> w519
            tunnel: w500 -> [_ _]
            frame False {
            }
            frame True {
              n184 = feedback #7(i32[] [0, 1]) -> (w529:i32[])
              n185 = feedback-in #7(w526) -> ()
              n186 = Increment(x=w529) -> (x+1=w528:i32[])
              n187 = Equal?(x=w528, y=w526) -> (x = y?=w527:bool)
            }
          }
          n188 = Compound Arithmetic op=AND(w522, w521) -> (w520:bool)
          n189 = Equal?(x=i32[] [10, 11], y=w519) -> (x = y?=w518:bool)
          n190 = Compound Arithmetic op=OR(w518, w505) -> (w517:bool)
        }
        n191 = while {
          tunnel: w487 -> [w531]
          shift-right: [w536] -> w493
          shift-left: w486 -> [w542]
          shift-right: [w533] -> _
          shift-left: i32[] [1, 2] -> [w534]
          tunnel: [w533] -> w475 mode=indexing if=w532
          tunnel: [w531] -> w488
          stop <- w535 stop-if-true
          n192 = call "Check Buffer Space Backpressure.vim"("error in (no error)"=w542, "Timeout (ns)"=i64 1000000, "CIPC BP References in"=w531) -> ("error out"=w541:errorcluster, "Timeout"=w539:bool, "CIPC Reference out"=w540:u64)  [unwired: 6 in]
          n193 = case shown="False" w539 {
            tunnel: w540 -> [w548 _]
            tunnel: w541 -> [w547 w551]
            tunnel: [w546 w551] -> w536
            tunnel: w534 -> [w545 w550]
            tunnel: [w544 w550] -> w533
            tunnel: [TRUE _] -> w532
            frame False {
              n194 = call "Write Element.vim"("error in (no error)"=w547, "Write Configuration"=T1 {"Prepend Array Size"=FALSE, "Get Write Position"=FALSE, "Notify Readers"=TRUE}, "Data in"=w545, "CIPC Reference in"=w548) -> ("error out"=w546:errorcluster)  [unwired: 4 in, 3 out]
              n195 = Increment(x=w545) -> (x+1=w544:i32[])
            }
            frame True {
              # "Timeout"
            }
          }
          n196 = Equal?(x=w533, y=i32[] [11, 12]) -> (x = y?=w537:bool)
          n197 = Compound Arithmetic op=OR(w537, w536) -> (w535:bool)
        }
        n198 = Index Array(array=w475, index (col)=0 ("disabled index (col)")) -> (element=w474:i32[])  [unwired: 1 in]
        n199 = Array Size(array=w474) -> (size(s)=w480:i32)
        n200 = Index Array(array=w473, index (col)=0 ("disabled index (col)")) -> (element=w472:i32[])  [unwired: 1 in]
        n201 = Merge Errors(w493, w494) -> (w495:errorcluster)
        n202 = Equal?(x=w480, y=10 ("x")) -> (x = y?=w478:bool)
        n203 = Array Size(array=w472) -> (size(s)=w485:i32)
        n204 = Equal?(x=10, y=w485) -> (x = y?=w482:bool)
        n205 = call "Close Backpressure.vi"("error in (no error)"=w495, "CIPC BP References in"=w488) -> ("error out"=w489:errorcluster)  [unwired: 9 in]
        n206 = Compound Arithmetic op=AND(w478, w483, w482) -> (w481:bool)
        n207 = case shown="True" w481 {
          tunnel: w499 -> [w555 w556]
          tunnel: [w552 w556] -> w498
          tunnel: "Failed advanced partial read" -> [w554 _]
          tunnel: "\r" -> [w553 _]
          frame False {
            n208 = Concatenate Strings(w555, w554, w553) -> (w552:string)
          }
          frame True {
          }
        }
      }
    }
  }
  "error out" <- w2
  "status" <- w1
  n209 = And Array Elements(Boolean array=w7) -> (logical AND=→"pass":bool)
